vi "CreateDataReqPacket.vi"(7 "SequenceNumber":u32) -> (3 "DataReqPacket":string)   [LabVIEW 2009]
panel:
  out "FCP Packet":u32[](array[numeric])
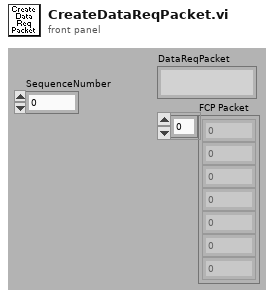
[diagram p1: front panel]
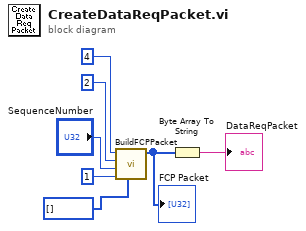
[diagram p0: block diagram]
diagram:
  n1 = call "BuildFCPPacket.vi"("Data"=u32[] [], "Data Length (in Bytes)"=1, "SequenceNumber"="SequenceNumber", "Channel"=2, "Command"=4) -> ("FCP Packet"=w2:u32[])  [unwired: 6 in]
  "FCP Packet" <- w2
  n2 = Byte Array To String(unsigned byte array=w2) -> (string=→"DataReqPacket":string)
